vi "Minerva subsys.vi"(4 "GB":cluster{dbl, dbl, dbl[], dbl[]}, 5 "nu_c_ned":dbl[](array[numeric])=[0.0, 0.0, 0.0, 0.0, 0.0, 0.0], 6 "tau":dbl[](array[numeric])=[0.0, 0.0, 0.0, 0.0, 0.0, 0.0], 7 "MD":T1) -> (0 "nu_dot":dbl[](array[numeric]), 1 "nu":dbl[](array[numeric]), 2 "nu_r":dbl[](array[numeric]), 3 "eta":dbl[](array[numeric]))   [LabVIEW 2014]
uses:
  <vilib>/Simulation/Implementation/Shared/SIMSCR Execution Mode.ctl
  <vilib>/Simulation/Scripting/Companion Diagram/SimConfigNode/SimParams.ctl
  <vilib>/Simulation/Scripting/Companion Diagram/SimConfigNode/_simSolvers.ctl
  <vilib>/Simulation/Param Hierarchy/Typedefs/SIMPH Param Control Actions.ctl
  <vilib>/Simulation/Implementation/Shared/SIM limit type.ctl
  <vilib>/Simulation/Implementation/Shared/NILVSim_ParamChanged.vi
  <vilib>/Simulation/Implementation/Shared/NILVSIM_BeginStep.vi
  <vilib>/Simulation/ContinuousLinear/Implementation/NILVSim Integrator new.llb/SIM Integrator Distributor (vector).vi
  <vilib>/Simulation/SignalArithmetic/Implementation/NILVSim Gain.llb/SIM Gain (vector,MatrixGain).vi
  <vilib>/Simulation/ContinuousLinear/Implementation/NILVSim Integrator new.llb/SIM Integrator Collector (vector).vi
  <vilib>/Simulation/Implementation/Shared/NILVSim_Manager.vi
  <vilib>/Utility/error.llb/Clear Errors.vi
  <vilib>/Simulation/Implementation/Shared/NILVSim_FinalizeModel.vi
  <vilib>/Simulation/Implementation/Shared/SIM Unbundle Sim Info.vi
  <vilib>/Simulation/Implementation/Shared/SIMSH Read Queue.vi
  <vilib>/Simulation/Implementation/Shared/NILVSim_Initialize.vi
  <vilib>/imath/engines/lvmath2/RunTimeEngine/IndexRead/NIMS V(R2).vi
  <instcachedir>/0/NIMS V(R2)_C76619605A0E4E9F8B2FA9389712AC47.lvgen/NIMS V(R2)_C76619605A0E4E9F8B2FA9389712AC47_000.vi
  <vilib>/imathl/engines/lvmath/Functions/Error Handling/Create Error.vi
  <vilib>/imath/engines/lvmath2/RunTimeEngine/ArithmeticOperatorToken/NIMS_ArithmeticOperator_plus.vi
  <instcachedir>/0/NIMS_ArithmeticOperator_plus_48D6EAACA5D645B09F7EC9C016C2DEA8.lvgen/NIMS_ArithmeticOperator_plus_48D6EAACA5D645B09F7EC9C016C2DEA8_003.vi
  <vilib>/imath/engines/lvmath2/RunTimeEngine/IndexRead/NIMS M(R2,R2).vi
  <instcachedir>/0/NIMS M(R2,R2)_A604CBC2A3B94D18B31C03B21D5CD7AA.lvgen/NIMS M(R2,R2)_A604CBC2A3B94D18B31C03B21D5CD7AA_000.vi
  <vilib>/imath/engines/lvmath2/RunTimeEngine/ArithmeticOperatorToken/NIMS_ArithmeticOperator_multmx(M,CV)-internal.vi
  <instcachedir>/0/NIMS_ArithmeticOperator_multmx(M,CV)-internal_25C7CE5937BA4322B5BE2717374345EA.lvgen/NIMS_ArithmeticOperator_multmx(M,CV)-internal_25C7CE5937BA4322B5BE2717374345EA_001.vi
  <vilib>/imath/engines/lvmath2/RunTimeEngine/ErrorHandling/NIMS_Create Error From Enums.vi
  <vilib>/imath/engines/lvmath2/RunTimeEngine/IndexRead/NIMS V(S).vi
  <instcachedir>/0/NIMS V(S)_0488751826AF41519A22953C041130DC.lvgen/NIMS V(S)_0488751826AF41519A22953C041130DC_000.vi
  <vilib>/imath/engines/lvmath2/RunTimeEngine/RowToken/NIMS_RowToken_M_M.vi
  <instcachedir>/0/NIMS_RowToken_M_M_4C96C156B57B4BCFA08E125188784392.lvgen/NIMS_RowToken_M_M_4C96C156B57B4BCFA08E125188784392_004.vi
  <vilib>/imath/engines/lvmath2/RunTimeEngine/NodeEndStatement/NIMS_NodeEndStatement_Output.vi
  <instcachedir>/0/NIMS_NodeEndStatement_Output_53EC0D466D134D7ABD903AC30B43404B.lvgen/NIMS_NodeEndStatement_Output_53EC0D466D134D7ABD903AC30B43404B_002.vi
  <vilib>/imath/engines/lvmath2/RunTimeEngine/ErrorHandling/NIMS_Finalize Error.vi
  <vilib>/imath/engines/lvmath2/RunTimeEngine/ArithmeticOperatorToken/NIMS_ArithmeticOperator_multmx(M,CV).vi
  <instcachedir>/0/NIMS_ArithmeticOperator_multmx(M,CV)_787B4652E60B4C52835A7FB23671E425.lvgen/NIMS_ArithmeticOperator_multmx(M,CV)_787B4652E60B4C52835A7FB23671E425_000.vi
  <vilib>/imath/engines/lvmath2/RunTimeEngine/NodeEndStatement/NIMS_NodeEndStatement_Get Vector.vi
  <instcachedir>/0/NIMS_NodeEndStatement_Get Vector_00D1625602D843AD9D7EC134A9EC13A2.lvgen/NIMS_NodeEndStatement_Get Vector_00D1625602D843AD9D7EC134A9EC13A2_001.vi
  <instcachedir>/0/NIMS_NodeEndStatement_Output_53EC0D466D134D7ABD903AC30B43404B.lvgen/NIMS_NodeEndStatement_Output_53EC0D466D134D7ABD903AC30B43404B_005.vi
  <vilib>/imath/engines/lvmath/Functions/Error Handling/MergeErrorsWrapper.vi
  <vilib>/Simulation/Utility/Implementation/NILVSim Get Time and IsAcceptedStep.vi
  <vilib>/Simulation/Implementation/Shared/NILVSim_GetModelError.vi
  <vilib>/Simulation/Implementation/Shared/SIM SimErrorHandler.vi
  <vilib>/Simulation/Implementation/Shared/SIM Bundle Sim Info.vi
  <vilib>/Simulation/Scripting/Companion Diagram/SimConfigNode/SimDog.xnode
  <vilib>/Simulation/Implementation/XNodeFramework/SimXNode/SimX.xnode
  <vilib>/Simulation/ContinuousLinear/Implementation/NILVSim Integrator new.llb/SIM Integrator (vector).vi
  <vilib>/Simulation/Implementation/Shared/NI_SIM_Implementation.lvlib
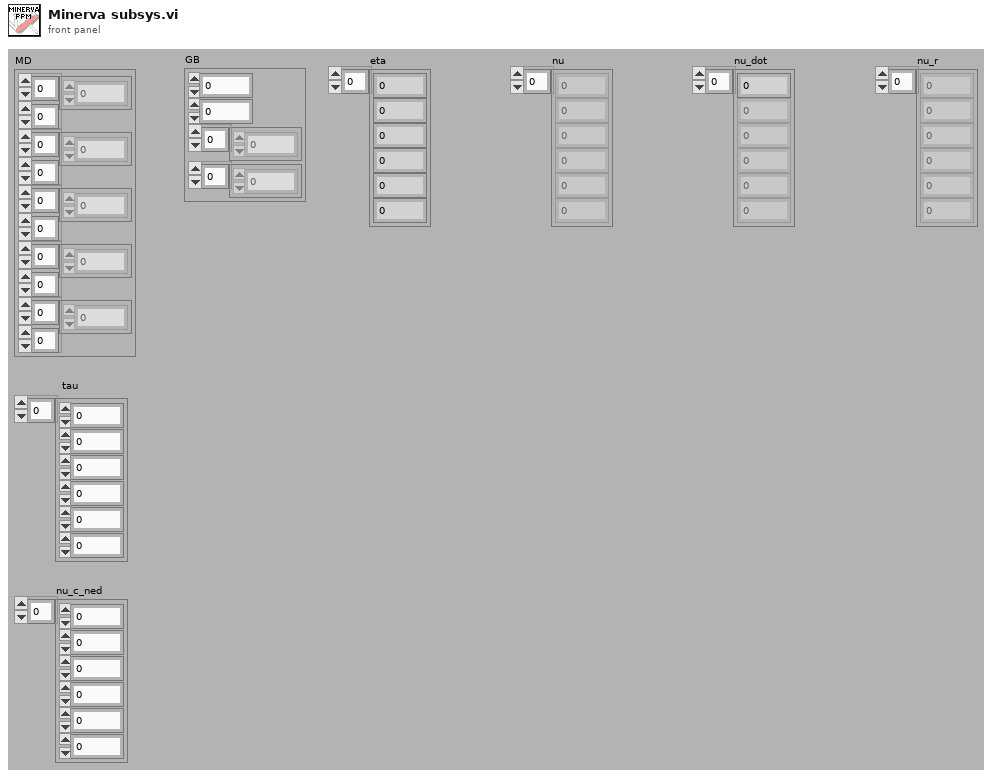
[diagram p1: front panel]
types:
  T1 = cluster{dbl[][], dbl[][], dbl[][], dbl[][], dbl[][]}
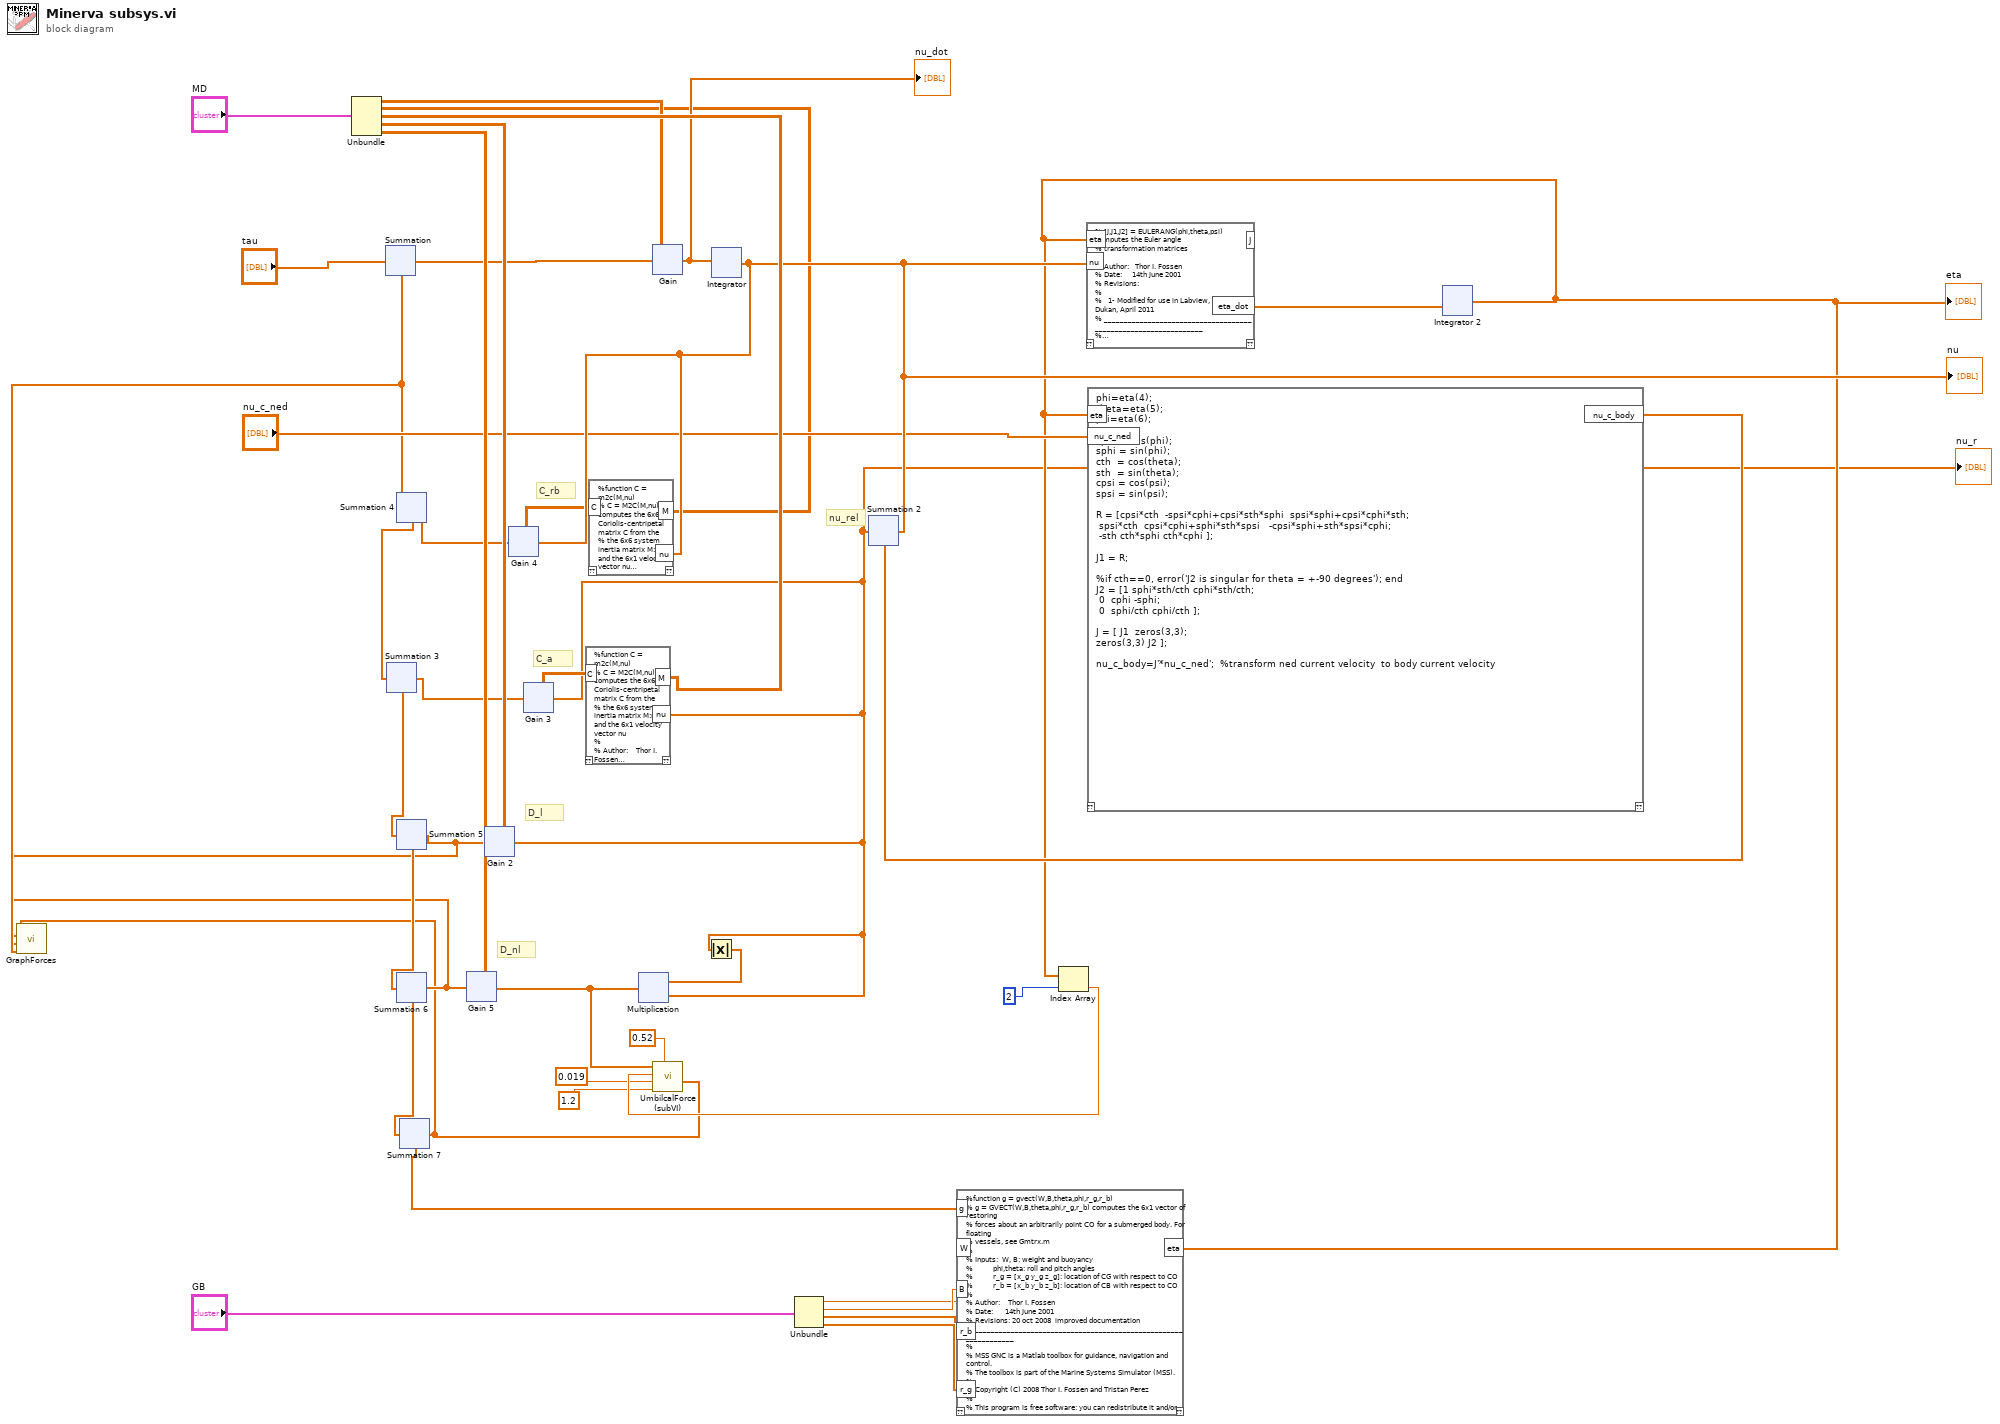
[diagram p0: block diagram]
diagram:
  # "D_nl"
  # "D_l"
  # "C_a"
  # "C_rb"
  # "nu_rel"
  n1 = Unbundle("MD") -> (w32:dbl[][], w15:dbl[][], w33:dbl[][], w34:dbl[][], w35:dbl[][])
  n2 = Unbundle ("Unbundle 2")("GB") -> (w37:dbl, w38:dbl, w39:dbl[], w40:dbl[])
  n3 = call "GraphForces.vi"("Tot envir"=w4, "D_L"=w3, "D_NL"=w2, "Umbilical"=w1) -> ()  [unwired: 8 in]
  n4 = xnode ("Summation")("Operand1"="tau", "Operand2"=w4) -> ("Result"=w17:dbl[])
  n5 = xnode ("Gain")("gain"=w32, "input"=w17) -> ("output"=w18:dbl[])  [unwired: 2 in]
  "nu_dot" <- w18
  n6 = xnode ("Integrator")("input"=w18) -> ("output"=w26:dbl[])  [unwired: 9 in, 2 out]
  "nu" <- w26
  n7 = mathscript code="%function C = m2c(M,nu)\n% C = M2C(M,nu) computes the 6x6 Coriolis-centripetal matrix C from the\n% the 6x6 system inertia matrix M>0 and the 6x1 velocity vector nu \n% \n% Author:    Thor I. Fossen\n% Date:      14th June 2001\n% Revisions: 26th June 2002,  M21 = M12 is corrected to M12'\n%            10th Jan 2004, the computation of C is generalized to a nonsymmetric M > 0\n% ________________________________________________________________\n%\n% MSS GNC is a Matlab toolbox for guidance, navigation and control.\n% The toolbox is part of the Marine Systems Simulator (MSS).\n%\n% Copyright (C) 2008 Thor I. Fossen and Tristan Perez\n% \n% This program is free software: you can redistribute it and/or modify\n% it under the terms of the GNU General Public License as published by\n% the Free Software Foundation, either version 3 of the License, or\n% (at your option) any later version.\n% \n% This program is distributed in the hope that it will be useful, but\n% WITHOUT ANY WARRANTY; without even the implied warranty of\n% MERCHANTABILITY or FITNESS FOR A PARTICULAR PURPOSE.  See the \n% GNU General Public License for more details.\n% \n% You should have received a copy of the GNU General Public License\n% along with this program.  If not, see <http://www.gnu.org/licenses/>.\n% \n% E-mail: contact@marinecontrol.org\n% URL:    <http://www.marinecontrol.org>\n\nnu=nu';\n\nnu1 = nu(1:3);\nnu2 = nu(4:6);\n\n% T = 1/2 (v'Mv) = 1/2 v'(1/2(M + M')+1/2(M-M')) v =  1/2 v' Msym v\n% Msym = 1/2 (M+M')\n\nMsym = 0.5*(M+M');\nM = Msym;\n\nM11 = M(1:3,1:3);\nM12 = M(1:3,4:6);\nM21 = M12';\nM22 = M(4:6,4:6);\n\ndt_dnu1 = M11*nu1 + M12*nu2;\ndt_dnu2 = M21*nu1 + M22*nu2;\n\nS1 = [    0  -dt_dnu1(3)   dt_dnu1(2);\n      dt_dnu1(3)     0   -dt_dnu1(1);\n     -dt_dnu1(2)   dt_dnu1(1)     0 ];\n\nS2 = [    0  -dt_dnu2(3)   dt_dnu2(2);\n      dt_dnu2(3)     0   -dt_dnu2(1);\n     -dt_dnu2(2)   dt_dnu2(1)     0 ];\n\nC = [ zeros(3,3)   -S1;\n      -S1  -S2 ];" ("MathScript Node 4")("nu"=w26, "M"=w15) -> ("C"=w25:dbl[][])  [unwired: 1 in, 1 out]
  n8 = xnode ("Gain 4")("gain"=w25, "input"=w26) -> ("output"=w27:dbl[])  [unwired: 2 in]
  n9 = xnode ("Summation 3")("Operand1"=w24, "Operand2"=w29) -> ("Result"=w22:dbl[])
  n10 = xnode ("Summation 4")("Operand1"=w27, "Operand2"=w22) -> ("Result"=w4:dbl[])
  n11 = xnode ("Summation 5")("Operand1"=w3, "Operand2"=w30) -> ("Result"=w29:dbl[])
  n12 = xnode ("Summation 6")("Operand1"=w2, "Operand2"=w5) -> ("Result"=w30:dbl[])
  n13 = xnode ("Summation 7")("Operand1"=w1, "Operand2"=w6) -> ("Result"=w5:dbl[])
  n14 = xnode ("Gain 5")("gain"=w35, "input"=w14) -> ("output"=w2:dbl[])  [unwired: 2 in]
  n15 = xnode ("Gain 2")("gain"=w34, "input"=w7) -> ("output"=w3:dbl[])  [unwired: 2 in]
  n16 = xnode ("Gain 3")("gain"=w23, "input"=w7) -> ("output"=w24:dbl[])  [unwired: 2 in]
  n17 = mathscript code="%function C = m2c(M,nu)\n% C = M2C(M,nu) computes the 6x6 Coriolis-centripetal matrix C from the\n% the 6x6 system inertia matrix M>0 and the 6x1 velocity vector nu \n% \n% Author:    Thor I. Fossen\n% Date:      14th June 2001\n% Revisions: 26th June 2002,  M21 = M12 is corrected to M12'\n%            10th Jan 2004, the computation of C is generalized to a nonsymmetric M > 0\n% ________________________________________________________________\n%\n% MSS GNC is a Matlab toolbox for guidance, navigation and control.\n% The toolbox is part of the Marine Systems Simulator (MSS).\n%\n% Copyright (C) 2008 Thor I. Fossen and Tristan Perez\n% \n% This program is free software: you can redistribute it and/or modify\n% it under the terms of the GNU General Public License as published by\n% the Free Software Foundation, either version 3 of the License, or\n% (at your option) any later version.\n% \n% This program is distributed in the hope that it will be useful, but\n% WITHOUT ANY WARRANTY; without even the implied warranty of\n% MERCHANTABILITY or FITNESS FOR A PARTICULAR PURPOSE.  See the \n% GNU General Public License for more details.\n% \n% You should have received a copy of the GNU General Public License\n% along with this program.  If not, see <http://www.gnu.org/licenses/>.\n% \n% E-mail: contact@marinecontrol.org\n% URL:    <http://www.marinecontrol.org>\n\nnu=nu';\n\nnu1 = nu(1:3);\nnu2 = nu(4:6);\n\n% T = 1/2 (v'Mv) = 1/2 v'(1/2(M + M')+1/2(M-M')) v =  1/2 v' Msym v\n% Msym = 1/2 (M+M')\n\nMsym = 0.5*(M+M');\nM = Msym;\n\nM11 = M(1:3,1:3);\nM12 = M(1:3,4:6);\nM21 = M12';\nM22 = M(4:6,4:6);\n\ndt_dnu1 = M11*nu1 + M12*nu2;\ndt_dnu2 = M21*nu1 + M22*nu2;\n\nS1 = [    0  -dt_dnu1(3)   dt_dnu1(2);\n      dt_dnu1(3)     0   -dt_dnu1(1);\n     -dt_dnu1(2)   dt_dnu1(1)     0 ];\n\nS2 = [    0  -dt_dnu2(3)   dt_dnu2(2);\n      dt_dnu2(3)     0   -dt_dnu2(1);\n     -dt_dnu2(2)   dt_dnu2(1)     0 ];\n\nC = [  zeros(3,3)      -S1;\n      -S1  -S2 ];" ("MathScript Node 5")("nu"=w7, "M"=w33) -> ("C"=w23:dbl[][])  [unwired: 1 in, 1 out]
  n18 = xnode ("Multiplication")("Operand1"=w28, "Operand2"=w7) -> ("Result"=w14:dbl[])
  n19 = call "UmbilcalForce (subVI).vi"("r_z"=0.52 ("Constant 4"), "Drag Coeffecient"=1.2 ("Constant 3"), "Diameter"=0.019 ("Constant 2"), "Depth"=w11, "Velocity"=w14) -> ("Forces"=w1:dbl[])  [unwired: 6 in]
  n20 = Absolute Value(x=w7) -> (abs(x)=w28:dbl[])
  n21 = xnode ("Summation 2")("Operand1"=w26, "Operand2"=w21) -> ("Result"=w7:dbl[])
  "nu_r" <- w7
  n22 = mathscript code="%function g = gvect(W,B,theta,phi,r_g,r_b)\n% g = GVECT(W,B,theta,phi,r_g,r_b) computes the 6x1 vector of restoring \n% forces about an arbitrarily point CO for a submerged body. For floating \n% vessels, see Gmtrx.m\n% \n% Inputs:  W, B: weight and buoyancy\n%          phi,theta: roll and pitch angles\n%          r_g = [x_g y_g z_g]: location of CG with respect to CO\n%          r_b = [x_b y_b z_b]: location of CB with respect to CO\n%\n% Author:    Thor I. Fossen\n% Date:      14th June 2001\n% Revisions: 20 oct 2008  improved documentation\n% ________________________________________________________________\n%\n% MSS GNC is a Matlab toolbox for guidance, navigation and control.\n% The toolbox is part of the Marine Systems Simulator (MSS).\n%\n% Copyright (C) 2008 Thor I. Fossen and Tristan Perez\n% \n% This program is free software: you can redistribute it and/or modify\n% it under the terms of the GNU General Public License as published by\n% the Free Software Foundation, either version 3 of the License, or\n% (at your option) any later version.\n% \n% This program is distributed in the hope that it will be useful, but\n% WITHOUT ANY WARRANTY; without even the implied warranty of\n% MERCHANTABILITY or FITNESS FOR A PARTICULAR PURPOSE.  See the \n% GNU General Public License for more details.\n% \n% You should have received a copy of the GNU General Public License\n% along with this program.  If not, see <http://www.gnu.org/licenses/>.\n% \n% E-mail: contact@marinecontrol.org\n% URL:    <http://www.marinecontrol.org>\n\nphi=eta(4);\ntheta=eta(5);\npsi=eta(6);\n\nsth  = sin(theta); cth  = cos(theta);\nsphi = sin(phi);   cphi = cos(phi);\n\ng = [(W-B)*sth;\n  -(W-B)*cth*sphi;\n  -(W-B)*cth*cphi;\n  -(r_g(2)*W-r_b(2)*B)*cth*cphi + (r_g(3)*W-r_b(3)*B)*cth*sphi;\n   (r_g(3)*W-r_b(3)*B)*sth      + (r_g(1)*W-r_b(1)*B)*cth*cphi;\n  -(r_g(1)*W-r_b(1)*B)*cth*sphi + (r_g(2)*W-r_b(2)*B)*sth];"("eta"=w13, "W"=w37, "B"=w38, "r_b"=w39, "r_g"=w40) -> ("g"=w6:dbl[])  [unwired: 1 in, 1 out]
  n23 = Index Array(array=w13, index=2 ("Constant")) -> (element=w11:dbl)
  n24 = mathscript code="% [J,J1,J2] = EULERANG(phi,theta,psi) computes the Euler angle\n% transformation matrices\n%\n% Author:   Thor I. Fossen\n% Date:     14th June 2001\n% Revisions: \n%  \n%   1- Modified for use in Labview, Fredrik Dukan, April 2011\n% ________________________________________________________________\n%\n% MSS GNC is a Matlab toolbox for guidance, navigation and control.\n% The toolbox is part of the Marine Systems Simulator (MSS).\n%\n% Copyright (C) 2008 Thor I. Fossen and Tristan Perez\n% \n% This program is free software: you can redistribute it and/or modify\n% it under the terms of the GNU General Public License as published by\n% the Free Software Foundation, either version 3 of the License, or\n% (at your option) any later version.\n% \n% This program is distributed in the hope that it will be useful, but\n% WITHOUT ANY WARRANTY; without even the implied warranty of\n% MERCHANTABILITY or FITNESS FOR A PARTICULAR PURPOSE.  See the \n% GNU General Public License for more details.\n% \n% You should have received a copy of the GNU General Public License\n% along with this program.  If not, see <http://www.gnu.org/licenses/>.\n% \n% E-mail: contact@marinecontrol.org\n% URL:    <http://www.marinecontrol.org>\n\nphi=eta(4);\ntheta=eta(5);\npsi=eta(6);\n\ncphi = cos(phi);\nsphi = sin(phi);\ncth  = cos(theta);\nsth  = sin(theta);\ncpsi = cos(psi);\nspsi = sin(psi);\n\nR = [cpsi*cth  -spsi*cphi+cpsi*sth*sphi  spsi*sphi+cpsi*cphi*sth;\n spsi*cth  cpsi*cphi+sphi*sth*spsi   -cpsi*sphi+sth*spsi*cphi;\n -sth cth*sphi cth*cphi ];\n\nJ1 = R;\n\n%if cth==0, error('J2 is singular for theta = +-90 degrees'); end\nJ2 = [1 sphi*sth/cth cphi*sth/cth;\n 0  cphi -sphi;\n 0  sphi/cth cphi/cth ];\n\nJ = [ J1  zeros(3,3);\nzeros(3,3) J2 ];\n\neta_dot=J*nu';" ("MathScript Node 2")("nu"=w26, "eta"=w13) -> ("eta_dot"=w19:dbl[])  [unwired: 1 in, 2 out]
  n25 = xnode ("Integrator 2")("input"=w19) -> ("output"=w13:dbl[])  [unwired: 9 in, 2 out]
  "eta" <- w13
  n26 = mathscript code="phi=eta(4);\ntheta=eta(5);\npsi=eta(6);\n\ncphi = cos(phi);\nsphi = sin(phi);\ncth  = cos(theta);\nsth  = sin(theta);\ncpsi = cos(psi);\nspsi = sin(psi);\n\nR = [cpsi*cth  -spsi*cphi+cpsi*sth*sphi  spsi*sphi+cpsi*cphi*sth;\n spsi*cth  cpsi*cphi+sphi*sth*spsi   -cpsi*sphi+sth*spsi*cphi;\n -sth cth*sphi cth*cphi ];\n\nJ1 = R;\n\n%if cth==0, error('J2 is singular for theta = +-90 degrees'); end\nJ2 = [1 sphi*sth/cth cphi*sth/cth;\n 0  cphi -sphi;\n 0  sphi/cth cphi/cth ];\n\nJ = [ J1  zeros(3,3);\nzeros(3,3) J2 ];\n\nnu_c_body=J'*nu_c_ned';  %transform ned current velocity  to body current velocity" ("MathScript Node 3")("nu_c_ned"="nu_c_ned", "eta"=w13) -> ("nu_c_body"=w21:dbl[])  [unwired: 1 in, 1 out]
